vi "setSpectTempSetpoint.vi"(8 "error in (no error)":errorcluster, 9 "setSpectTempSetpoint":T1, 10 "CommandID":i32, 11 "IContextThisComponent in":refnum<class "IContextThisComponent.lvclass">) -> (0 "error out":errorcluster, 3 "IContextThisComponent out":refnum<class "IContextThisComponent.lvclass">)   [LabVIEW 2016, in "IContextThisComponent.lvclass"]
uses:
  IContextThisComponent.lvclass
  ts_sallv_sedspectrometer/DataTypes/command_setSpectTempSetpoint.ctl
  ts_sallv_sedspectrometer/SALLV_sedSpectrometer.lvlib
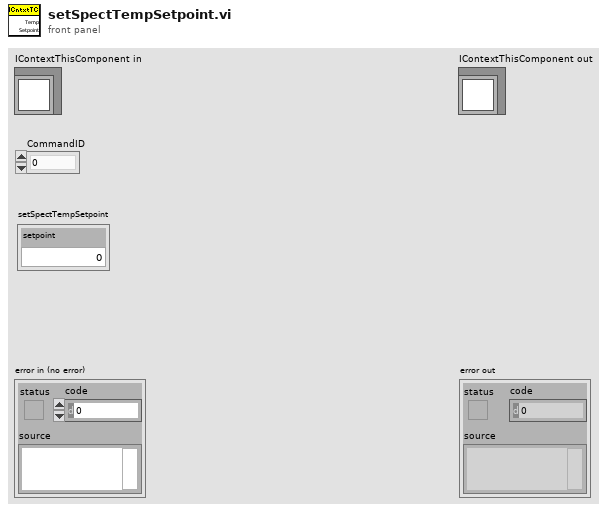
[diagram p1: front panel]
types:
  T1 = typedef "SALLV_sedSpectrometer.lvlib/command_setSpectTempSetpoint.ctl" = cluster{"setpoint":sgl}
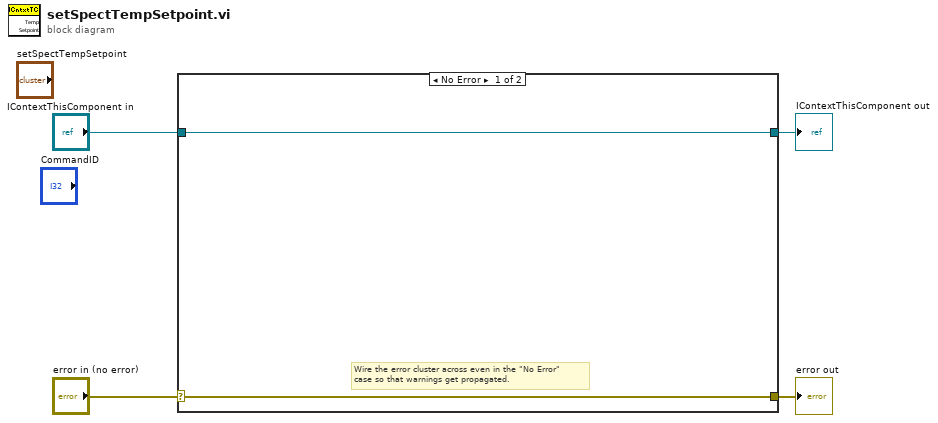
[diagram p0: block diagram]
diagram:
  n1 = case shown="No Error" "error in (no error)" {
    selector: "error in (no error)" -> [w5 w8]
    tunnel: [w5 w8] -> w3
    tunnel: [w6 w7] -> w1
    tunnel: "IContextThisComponent in" -> [w6 w7]
    frame No Error {
      # "Wire the error cluster across even in the \"No Error\"\ncase so that warnings get propagated."
    }
    frame Error {
    }
  }
  "error out" <- w3
  "IContextThisComponent out" <- w1
